vi "get_stocks.vi"   [LabVIEW 2023]
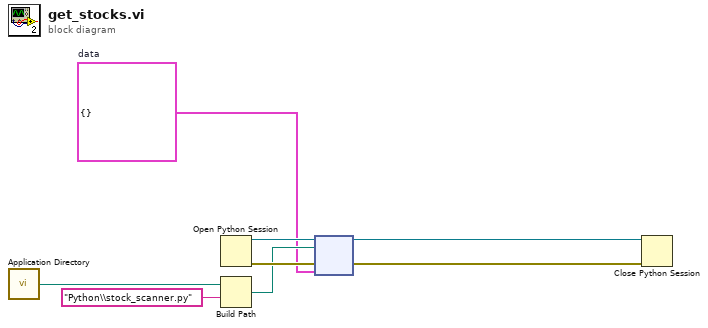
[diagram p0: block diagram]
diagram:
  w1 = cluster{} {}  # data
  n1 = call <vilib>:"Application Directory.vi"() -> ("Application Directory"=w4:path)
  n2 = Open Python Session() -> (session out=w8:refnum<k35>, error out=w7:errorcluster)  [unwired: 3 in]
  n3 = Build Path(base path=w4, name or relative path="Python\\stock_scanner.py") -> (appended path=w2:path)
  n4 = node(w8, w2, w7, w1) -> (w5:refnum<k35>, w6:errorcluster)  [unwired: 2 in, 2 out]
  n5 = Close Python Session(session in=w5, error in=w6) -> ()  [unwired: 1 out]
